vi "Wait for WriterState.vi"(8 "error in (no error)":errorcluster, 9 "timeout (5000 ms)":i32=5000, 11 "Target WriterState (T-Running/F-Idle)":bool) -> (0 "error out":errorcluster, 3 "timeout?":bool)   [LabVIEW 2021, in "XNET-CAN-Signal-Logger.lvlib"]
uses:
  XNET-CAN-Signal-Logger.lvlib
  Global Variables.vi
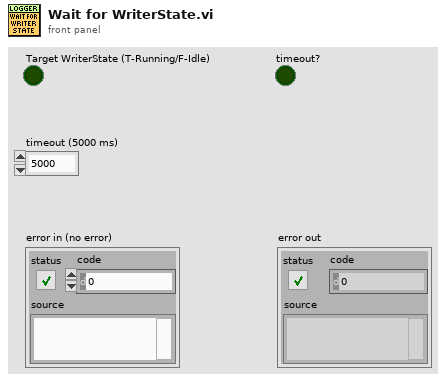
[diagram p1: front panel]
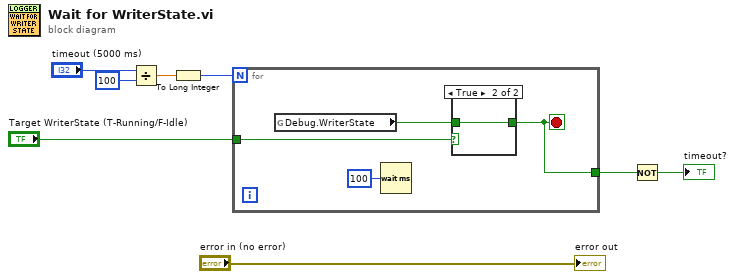
[diagram p0: block diagram]
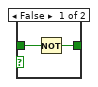
[diagram p2: hidden frame]
diagram:
  n1 = Divide(x="timeout (5000 ms)", y=100) -> (x/y=w3:dbl)
  n2 = To Long Integer(number=w3) -> (32bit integer=w1:i32)
  n3 = for {
    N: w1 -> [_]
    tunnel: [w10] -> w8
    tunnel: "Target WriterState (T-Running/F-Idle)" -> [w9]
    stop <- w10 stop-if-true
    n4 = global read "Global Variables.vi" "Debug.WriterState"() -> (w11:bool)
    n5 = Wait (ms)(milliseconds to wait=u32 100) -> ()  [unwired: 1 out]
    n6 = case shown="True" w9 {
      tunnel: w11 -> [w14 w15]
      tunnel: [w13 w15] -> w10
      frame False {
        n7 = Not(x=w14) -> (.not. x?=w13:bool)
      }
      frame True {
      }
    }
  }
  n8 = Not(x=w8) -> (.not. x?=→"timeout?":bool)
  "error out" <- "error in (no error)"
